vi "Configure Measurements (Integrator).vi"(8 "error in (no error)":errorcluster, 10 "Integrator Measurements":i32[](listbox)=[0, 1, 5, 6, 8], 11 "VISA resource name":refnum<visa-resource-name>) -> (0 "error out":errorcluster, 3 "VISA resource name out":refnum<visa-resource-name>)   [LabVIEW 2015, in "Voltech PM1000+.lvlib"]
doc: "Configures the measurement itmes, and return the selected measurement list and indicators. This vi is used when PM1000+ is set to Integrator mode by using \"Configure Mode\" vi."
uses:
  <instrlib>/Voltech PM1000+/Voltech PM1000+.lvlib
panel:
  # "Notice:  \nHold \"Ctrl\" key and click the \nmeasurements to select \nmultiple items."
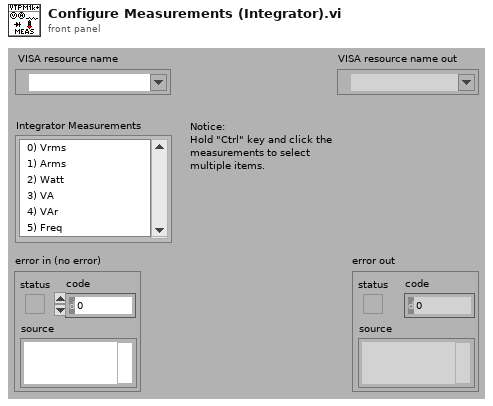
[diagram p1: front panel]
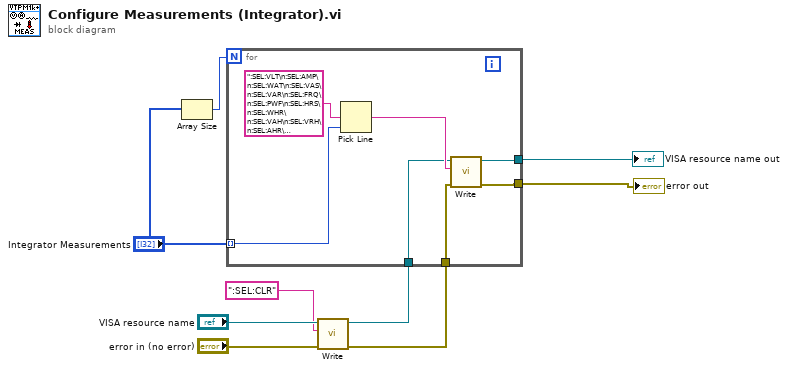
[diagram p0: block diagram]
diagram:
  n1 = Array Size(array="Integrator Measurements") -> (size(s)=w7:i32)
  n2 = call <instrlib>:"Write.vi"("error in (no error)"="error in (no error)", "Write Buffer"=":SEL:CLR" ("multi-line string"), "VISA resource name"="VISA resource name") -> ("error out"=w3:errorcluster, "VISA resource name out"=w4:refnum<visa-resource-name>)  [unwired: 7 in]
  n3 = for {
    N: w7 -> [_]
    tunnel: "Integrator Measurements" -> [w15] mode=indexing
    tunnel: [w11] -> w2
    tunnel: [w10] -> w1
    tunnel: w4 -> [w13]
    tunnel: w3 -> [w12]
    n4 = Pick Line(multi-line string=":SEL:VLT\n:SEL:AMP\n:SEL:WAT\n:SEL:VAS\n:SEL:VAR\n:SEL:FRQ\n:SEL:PWF\n:SEL:HRS\n:SEL:WHR\n:SEL:VAH\n:SEL:VRH\n:SEL:AHR\n:SEL:VRNG\n:SEL:ARNG", line index=w15) -> (output string=w14:string)  [unwired: 1 in]
    n5 = call <instrlib>:"Write.vi"("error in (no error)"=w12, "Write Buffer"=w14, "VISA resource name"=w13) -> ("error out"=w10:errorcluster, "VISA resource name out"=w11:refnum<visa-resource-name>)  [unwired: 7 in]
  }
  "error out" <- w1
  "VISA resource name out" <- w2
